vi "Get System Information.vi"(8 "error in":errorcluster, 11 "RT Management in":refnum<class "RT Management.lvclass">) -> (0 "error out":errorcluster, 2 "Network Device":T1={"System Hardware Reference"=refnum, "Device Information"={"Resource"="", "Vendor Name"="", "Product Name"="", "Product ID"=0, "Serial Number"="", "Device Class"="", "System Start Time"=timestamp(0 s since 1904-01-01), "Current Time"=timestamp(0 s since 1904-01-01), "Time Zone"="", "Firmware Revision"="", "Image Title"="", "Image Version"="", "System Status"="", "Credential type"=enum."None/Unlocked", "User Added"=FALSE}, "Primary Network Adapter"={"IP Address"="", "MAC Address"="", "IP Address Request Mode"=1, "SubnetMask"="", "Gateway"="", "DNS Server"="", "Adapter Mode"=1, "Adapter Type"=1}, "Secondary Network Adapters"=[]} {"Primary Network Adapter"."IP Address Request Mode" items=["Static"=1, "DHCP/Link Local"=2, "Link-Local Only"=4, "DHCP Only"=8]; "Primary Network Adapter"."Adapter Type" items=["Ethernet"=1, "WLAN"=2]; "Primary Network Adapter"."Adapter Mode" items=["Disabled"=1, "TCP/IP Ethernet"=2, "Deterministic"=4, "EtherCAT"=8, "TCP/IP WLAN Connect"=32, "TCP/IP WLAN Create"=64]; "Secondary Network Adapters"."IP Address Request Mode" items=["Static"=1, "DHCP/Link Local"=2, "Link-Local Only"=4, "DHCP Only"=8]; "Secondary Network Adapters"."Adapter Type" items=["Disabled"=1, "TCP/IP Ethernet"=2, "Deterministic"=4, "EtherCAT"=8, "TCP/IP WLAN Connect"=32, "TCP/IP WLAN Create"=64]; "Secondary Network Adapters"."Adapter Mode" items=["Disabled"=1, "TCP/IP Ethernet"=2, "Deterministic"=4, "EtherCAT"=8, "TCP/IP WLAN Connect"=32, "TCP/IP WLAN Create"=64]; "Device Information"."Product ID" format="%.0x"}, 3 "RT Management out":refnum<class "RT Management.lvclass">)   [LabVIEW 2015]
uses:
  RT Management.lvclass
  Distributed Devices/Controls/DeviceInformation.ctl
  Distributed Devices/Controls/NetworkAdapterSettings.ctl
  Distributed Devices/Controls/NetworkDevice.ctl
panel:
  in  "Network Adapters (F)":bool
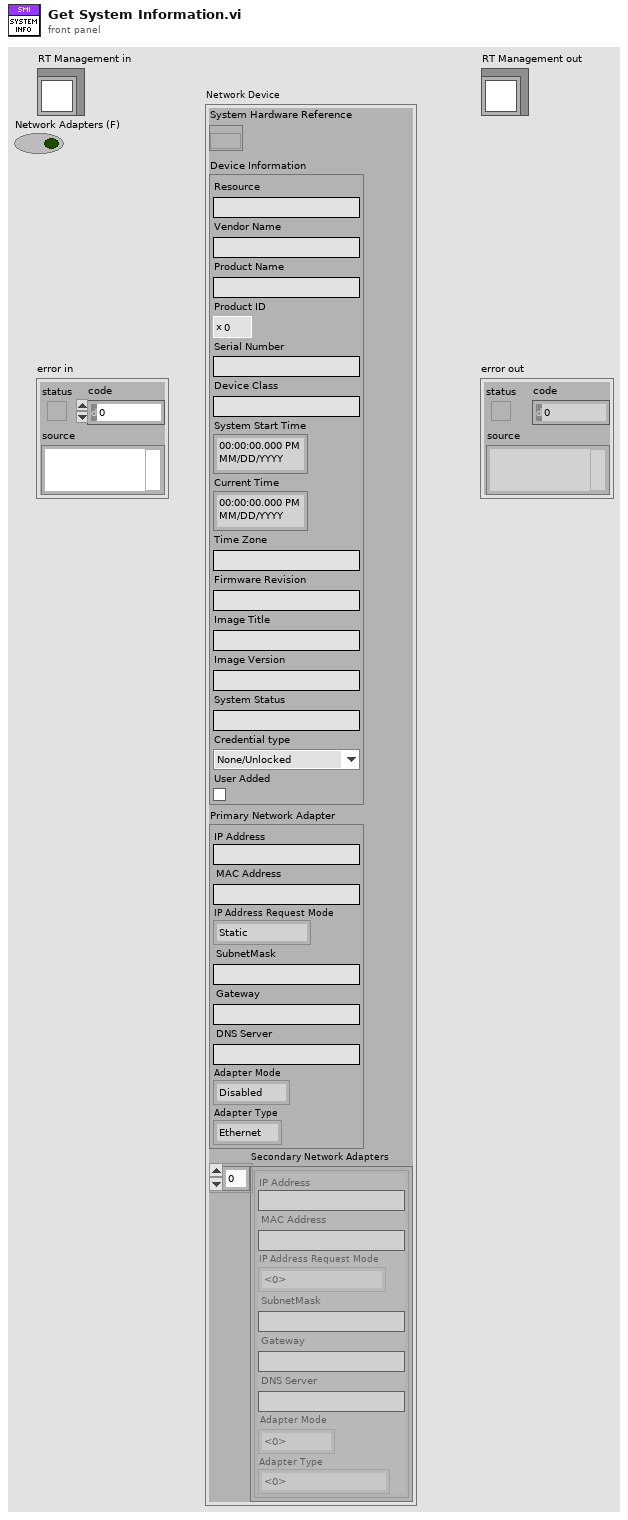
[diagram p1: front panel]
types:
  T1 = typedef "SMI.lvlib/Device.lvclass/NetworkDevice.ctl" = cluster{"System Hardware Reference":refnum<k20>, "Device Information":T2, "Primary Network Adapter":T3, "Secondary Network Adapters":T3[]}
  T2 = typedef "SMI.lvlib/Device.lvclass/DeviceInformation.ctl" = cluster{"Resource":string, "Vendor Name":string, "Product Name":string, "Product ID":u32, "Serial Number":string, "Device Class":string, "System Start Time":timestamp, "Current Time":timestamp, "Time Zone":string, "Firmware Revision":string, "Image Title":string, "Image Version":string, "System Status":string, "Credential type":enum16{"None/Unlocked", "FTP Password", "NIAuth Credentials"}, "User Added":bool}
  T3 = typedef "SMI.lvlib/Device.lvclass/NetworkAdapterSettings.ctl" = cluster{"IP Address":string, "MAC Address":string, "IP Address Request Mode":u32, "SubnetMask":string, "Gateway":string, "DNS Server":string, "Adapter Mode":u32, "Adapter Type":u32}
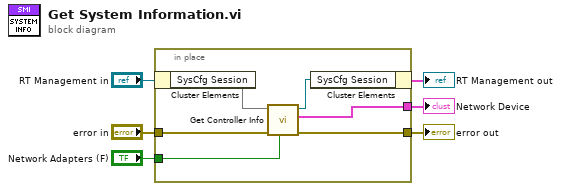
[diagram p0: block diagram]
diagram:
  n1 = in-place {
    in-place-border: "error in" -> [w12]
    in-place-border: [w11] -> w5
    in-place-border: [w10] -> w4
    in-place-border: "Network Adapters (F)" -> [w9]
    n2 = in-place-cluster #1("RT Management in") -> ("SysCfg Session"=w8)
    n3 = call "Get Controller Info.vi"("Network Adapters"=w9, "error in"=w12, "Session in"=w8) -> ("error out"=w11:errorcluster, "Network Device"=w10:T1, "Session out"=w7:refnum<k21>)  [unwired: 6 in]
    n4 = in-place-cluster #1("SysCfg Session"=w7) -> (→"RT Management out":cluster{})
  }
  "error out" <- w5
  "Network Device" <- w4
